vi "17-1.vi"() -> ()   [LabVIEW 2019, in "17.lvlib"]
uses:
  17.lvlib
panel:
  in  "Sample?":bool
  out "max Y":i32
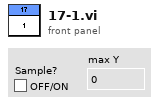
[diagram p1: front panel]
types:
  T1 = cluster{"x Velocity":i32, "Max Steps":i32, "Min Steps":i32, "Ignore Max":bool}[]
  T2 = cluster{"Tx min":i32, "Tx max":i32, "Ty min":i32, "Ty max":i32}
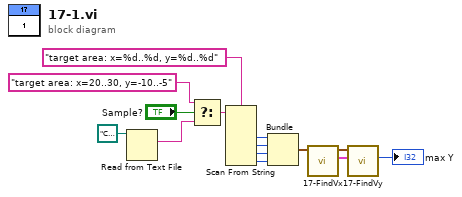
[diagram p0: block diagram]
diagram:
  n1 = Read from Text File(file (use dialog)=path "C:/Users/craig.walker/Documents/GitHub/lv2019-Advent-of-Code-2021/17/input.txt") -> (text=w10:string)  [unwired: 3 in, 3 out]
  n2 = Select(t="target area: x=20..30, y=-10..-5", s="Sample?", f=w10) -> (s? t:f=w12:string)
  n3 = Scan From String(format string="target area: x=%d..%d, y=%d..%d", input string=w12) -> (output 1=w6:i32, output 2=w5:i32, output 3=w4:i32, output 4=w3:i32)  [unwired: 6 in, 3 out]
  n4 = Bundle(w6, w5, w4, w3) -> (w2:cluster{i32, i32, i32, i32})  [unwired: 1 in]
  n5 = call "17-FindVx.vi"("Target in"=w2) -> ("x Velocity Info"=w8:T1, "Target out"=w7:T2)  [unwired: 9 in]
  n6 = call "17-FindVy.vi"("Vx"=w8, "Target"=w7) -> ("Max Y"=→"max Y":i32)  [unwired: 8 in, 1 out]
